vi "BottomPozition (SubVI).vi"(11 "Front Panel Window:Window Bounds":T1) -> (3 "Front Panel Window:Window Bounds 2":T1)   [LabVIEW 2017]
uses:
  <vilib>/Utility/miscctls.llb/LVRectTypeDef.ctl
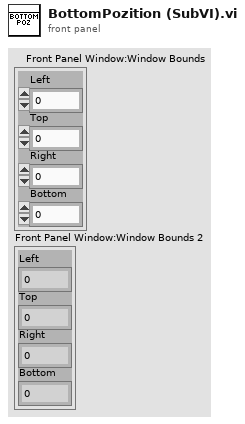
[diagram p1: front panel]
types:
  T1 = typedef "LVRectTypeDef.ctl" = cluster{"Left":i16, "Top":i16, "Right":i16, "Bottom":i16}
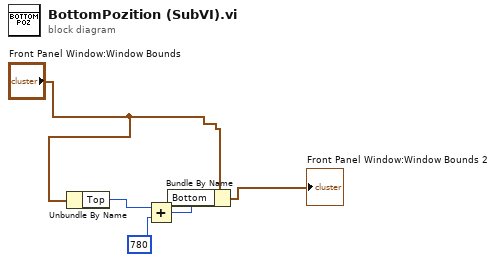
[diagram p0: block diagram]
diagram:
  n1 = Unbundle By Name("Front Panel Window:Window Bounds") -> ("Top"=w4:i16)
  n2 = Add(x=w4, y=i16 780) -> (x+y=w3:i16)
  n3 = Bundle By Name(cluster="Front Panel Window:Window Bounds", "Bottom"=w3) -> (→"Front Panel Window:Window Bounds 2":T1)
